vi "read_Rabi.vi"() -> (0 "fitted_signal":T2, 1 "fit_parameters":T4 {"mse" format="%.3g"; "T1" format="%.3g"; "C1" format="%.3g"; "Tm" format="%.3g"; "Cm" format="%.3g"; "Ie" format="%.3g"}, 2 "T1_curve":T3, 3 "T1_parameters":T1, 4 "file_path":path, 5 "timetags":u32[][](array[numeric]), 7 "triggers":u32[][](array[numeric]))   [LabVIEW 2014]
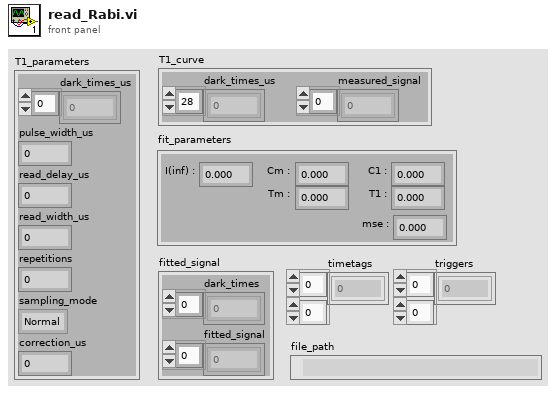
[diagram p1: front panel]
types:
  T1 = cluster{"dark_times_us":dbl[], "pulse_width_us":dbl, "read_delay_us":dbl, "read_width_us":dbl, "repetitions":i32, "sampling_mode":enum16{"Normal", "Sweep"}, "correction_us":dbl}
  T2 = cluster{"dark_times":dbl[], "fitted_signal":dbl[]}
  T3 = cluster{"dark_times_us":dbl[], "measured_signal":dbl[]}
  T4 = cluster{"Ie":dbl, "Cm":dbl, "Tm":dbl, "C1":dbl, "T1":dbl, "mse":dbl}
  T5 = enum16{"open", "replace", "create", "open or create", "replace or create", "replace or create with confirmation"}
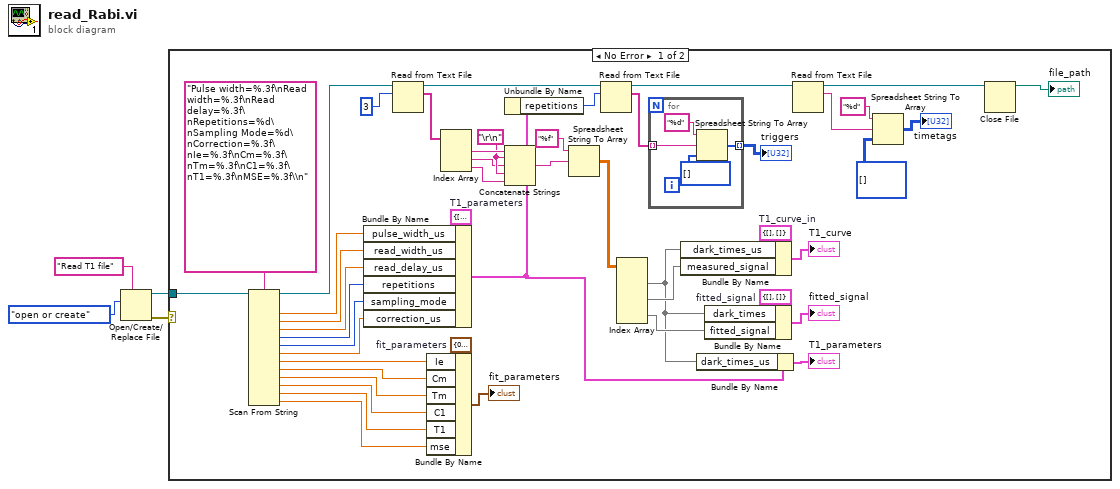
[diagram p0: block diagram]
diagram:
  n1 = Open/Create/Replace File(prompt="Read T1 file", operation (0:open)=T5."open or create") -> (refnum out=w1:refnum<file>, error out=w2:errorcluster)  [unwired: 4 in, 1 out]
  n2 = case shown="No Error" w2 {
    tunnel: w1 -> [w13 _]
    frame No Error {
      w18 = T1 {"dark_times_us"=[], "pulse_width_us"=0.0, "read_delay_us"=0.0, "read_width_us"=0.0, "repetitions"=0, "sampling_mode"=enum."Normal", "correction_us"=0.0}  # T1_parameters
      w21 = "\r\n"
      w35 = T3 {"dark_times_us"=[], "measured_signal"=[]}  # T1_curve_in
      w36 = T2 {"dark_times"=[], "fitted_signal"=[]}  # fitted_signal
      w46 = T4 {"Ie"=0.0, "Cm"=0.0, "Tm"=0.0, "C1"=0.0, "T1"=0.0, "mse"=0.0}  # fit_parameters
      n3 = Scan From String("Pulse width=%.3f\nRead width=%.3f\nRead delay=%.3f\nRepetitions=%d\nSampling Mode=%d\nCorrection=%.3f\nIe=%.3f\nCm=%.3f\nTm=%.3f\nC1=%.3f\nT1=%.3f\nMSE=%.3f\\n" ("format string"), w13) -> (w38:refnum<file>, output 1=w48:dbl, output 2=w49:dbl, output 3=w50:dbl, output 4=w51:i32, output 5=w17:i32, output 6=w16:dbl, output 7=w44:dbl, output 8=w43:dbl, output 9=w42:dbl, output 10=w41:dbl, output 11=w40:dbl, output 12=w39:dbl)  [unwired: 13 in, 1 out]
      n4 = Bundle By Name(cluster=w18, "pulse_width_us"=w48, "read_width_us"=w49, "read_delay_us"=w50, "repetitions"=w51, "sampling_mode"=w17, "correction_us"=w16) -> (w8:T1)
      n5 = Read from Text File(file (use dialog)=w38, count=3) -> (refnum out=w10:refnum<file>, text=w27:string[])  [unwired: 2 in, 2 out]
      n6 = Bundle By Name(cluster=w46, "Ie"=w44, "Cm"=w43, "Tm"=w42, "C1"=w41, "T1"=w40, "mse"=w39) -> (→"fit_parameters":T4)
      n7 = Index Array(array=w27) -> (element #1=w29:string, element #2=w20:string, element #3=w19:string)  [unwired: 3 in]
      n8 = Unbundle By Name(w8) -> ("repetitions"=w7:i32)
      n9 = Concatenate Strings(w29, w21, w20, w21, w19) -> (w26:string)
      n10 = Spreadsheet String To Array(format string="%f", spreadsheet string=w26) -> (array=w32:dbl[][])  [unwired: 2 in]
      n11 = Read from Text File(file (use dialog)=w10, count=w7) -> (refnum out=w9:refnum<file>, text=w6:string[])  [unwired: 2 in, 2 out]
      n12 = Index Array(array=w32) -> (element #1=w14:dbl[], element #2=w31:dbl[], element #3=w30:dbl[])  [unwired: 6 in]
      n13 = for {
        tunnel: w6 -> [w53] mode=indexing
        tunnel: [w52] -> w5 mode=indexing
        n14 = Spreadsheet String To Array(format string="%d", spreadsheet string=w53, array type (2D Dbl)=u32[] [] ("triggers")) -> (array=w52:u32[])  [unwired: 1 in]
      }
      "triggers" <- w5
      n15 = Bundle By Name(cluster=w35, "dark_times_us"=w14, "measured_signal"=w31) -> (→"T1_curve":T3)
      n16 = Bundle By Name(cluster=w8, "dark_times_us"=w14) -> (→"T1_parameters":T1)
      n17 = Bundle By Name(cluster=w36, "dark_times"=w14, "fitted_signal"=w30) -> (→"fitted_signal":T2)
      n18 = Read from Text File(file (use dialog)=w9) -> (refnum out=w12:refnum<file>, text=w24:string)  [unwired: 3 in, 2 out]
      n19 = Spreadsheet String To Array(format string="%d", spreadsheet string=w24, array type (2D Dbl)=u32[][] []) -> (array=→"timetags":u32[][])  [unwired: 1 in]
      n20 = Close File(refnum=w12) -> (path=→"file_path":path)  [unwired: 1 in, 1 out]
    }
    frame Error {
    }
  }
